vi "Write reference.vi"(8 "error in (no error)":errorcluster, 10 "reference":refnum<k24>, 11 "Abs Controler in":refnum<class "Abs Controler.lvclass">) -> (0 "error out":errorcluster, 3 "Abs Controler out":refnum<class "Abs Controler.lvclass">)   [LabVIEW 2020, in "HslCommunication.lvlib" / "Abs Controler.lvclass"]
uses:
  Abs Controler.lvclass
  E:/Git/Libraries/develop/PLCMonitor/HslCommunication/_Dependenciecs/HslCommunication.dll
  _Dependenciecs/HslCommunication.dll
  Abs Controler.lvclass/Abs Controler.ctl
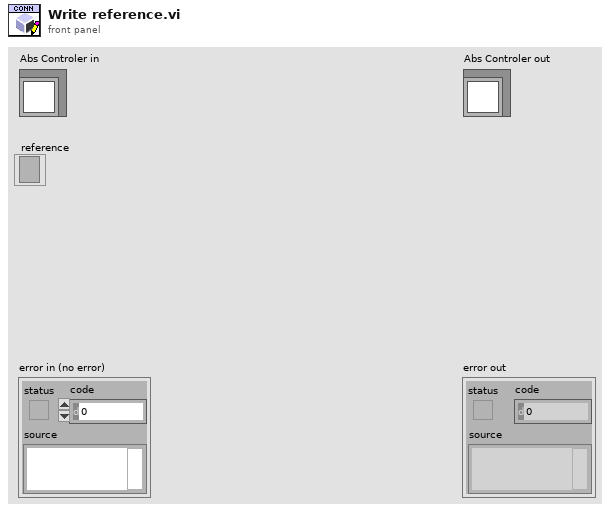
[diagram p1: front panel]
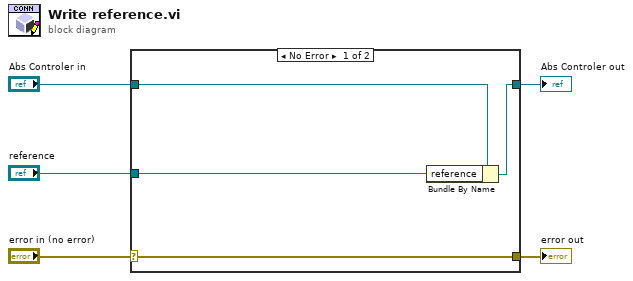
[diagram p0: block diagram]
diagram:
  n1 = case shown="No Error" "error in (no error)" {
    selector: "error in (no error)" -> [w9 w10]
    tunnel: [w9 w10] -> w4
    tunnel: [w7 w11] -> w2
    tunnel: "Abs Controler in" -> [w8 w11]
    tunnel: "reference" -> [w6 _]
    frame No Error {
      n2 = Bundle By Name(cluster=w8, "reference"=w6) -> (w7:refnum<class "Abs Controler.lvclass">)
    }
    frame Error {
    }
  }
  "error out" <- w4
  "Abs Controler out" <- w2
